vi "G#Object_GenericDefaultConstructor.vi"(0 "class path":path, 3 "control values":variant[](array[variant]), 4 "timeout in ms (-1)":i32=-1, 5 "error in (no error)":errorcluster) -> (14 "reference out":refnum<class "G#Object.lvclass">, 15 "external creator running?":bool, 19 "error out":errorcluster)   [LabVIEW 2017, in "G#Object.lvclass"]
doc: "Creates an instance of the class specified by the path by running the \"G#Object_Create.vi\" of the class. Override this construcor, else the default constructor runs. If the external create process is running, an event will be sent to let this process create and own the VI. This way LabVIEW garbage collector will not clear the object until it is destroyed or the garbage collector runs.\n\nBe careful when using this VI when building executables, since paths must be correct and make sure that all needed VIs are included in the build. Do not exclude unused dynamic dispatch VIs in the build script.\n\nNote: Will not work on RT systems."
uses:
  G#Object.lvclass
  utils/G#Object_EventType.ctl
  utils/G#Object_ObjectInfoType.ctl
  utils/G#Object_CreateMethod.ctl
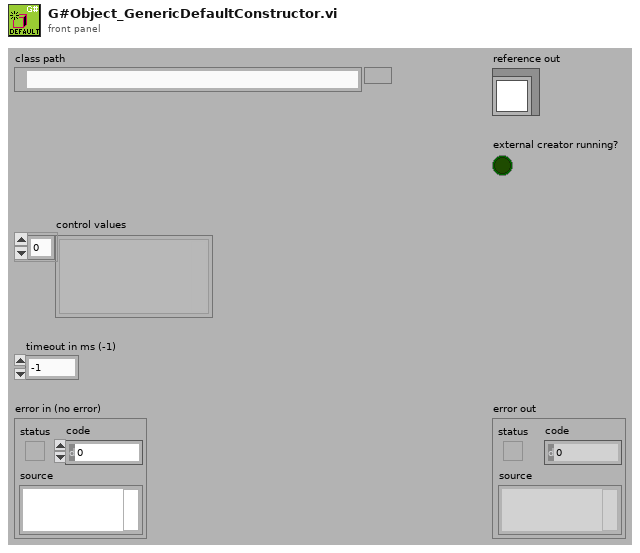
[diagram p1: front panel]
types:
  T1 = typedef "G#Object.lvclass/G#Object_ObjectInfoType.ctl" = cluster{"ObjectName":string, "ObjectID":u32, "Users":i32, "Counter":bool, "AttributeRefs":u32[], "FullClassName":string, "ClassName":string, "CreateMethod":T2, "GenericDestructorExists":bool, "Owner":string}
  T2 = typedef "G#Object.lvclass/G#Object_CreateMethod.ctl" = enum16{"Create", "Create or look up existing", "Look up existing"}
  T3 = typedef "G#Object.lvclass/G#Object_EventType.ctl" = enum16{"Created new", "Looked up existing", "Deleted", "Forced delete", "Not deleted", "Garbage collected", "Cleared", "User", "Error", "External create object", "External create class attributes", "Created class attributes", "Run constructor", "Run constructor done", "Run open method", "Run open method done"}
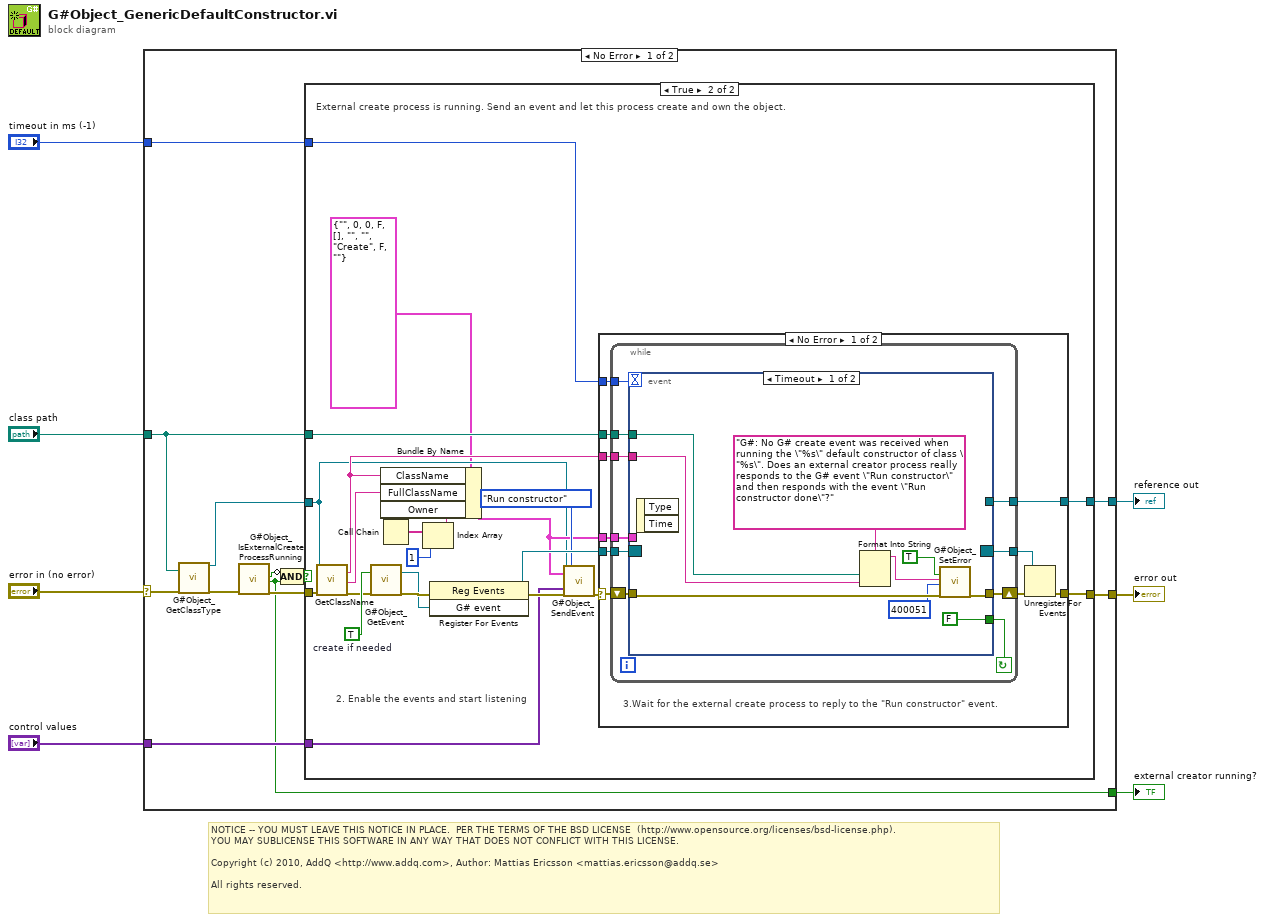
[diagram p0: block diagram]
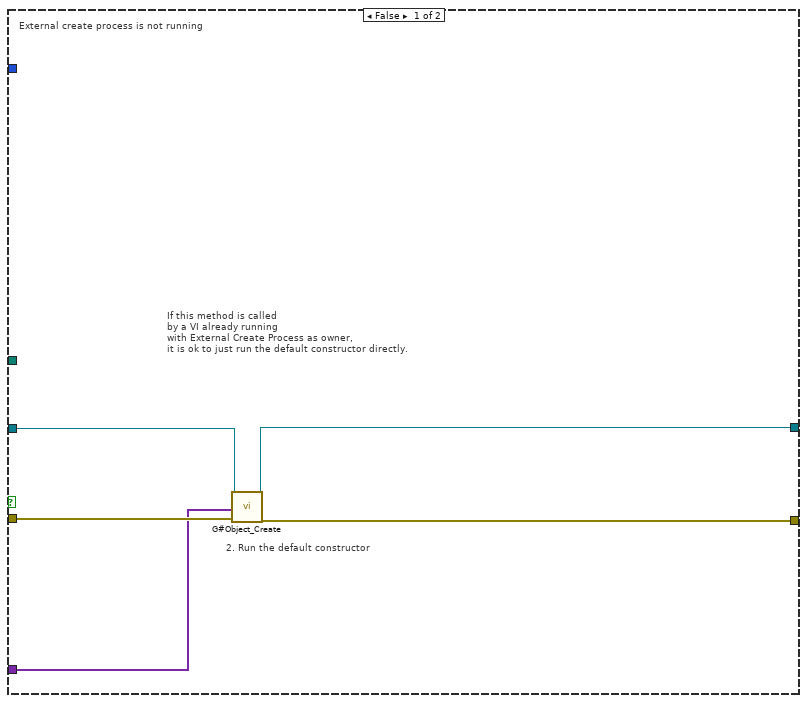
[diagram p2: hidden frame]
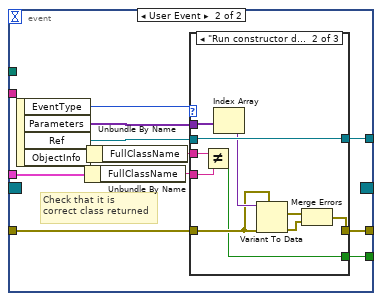
[diagram p3: hidden frame]
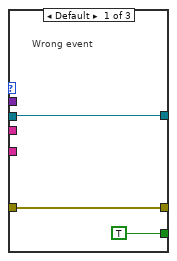
[diagram p4: hidden frame]
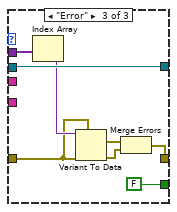
[diagram p5: hidden frame]
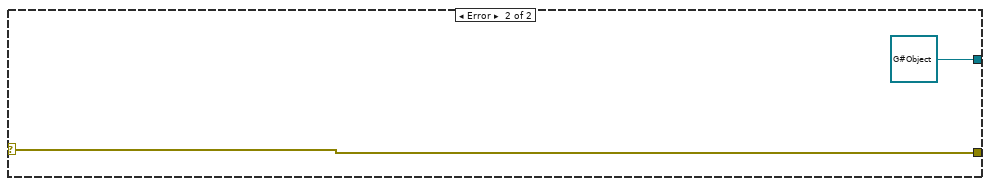
[diagram p7: hidden frame]
diagram:
  # "NOTICE -- YOU MUST LEAVE THIS NOTICE IN PLACE.  PER THE TERMS OF THE BSD LICENSE  (http://www.opensource.org/licenses/bsd-license.php).\nYOU MAY SUBLICENSE THIS SOFTWARE IN ANY WAY THAT DOES NOT CONFLICT WITH THIS LICENSE.\n\nCopyright (c) 2010, AddQ <http://www.addq.com>, Author: Mattias Ericsson <mattias.ericsson@addq.se>\n\nAll rights reserved."
  n1 = case shown="No Error" "error in (no error)" {
    selector: "error in (no error)" -> [w19 w110]
    tunnel: [w14 w110] -> w6
    tunnel: [w18 refnum<class "G#Object.lvclass"> refnum ("reference in (for type)")] -> w5
    tunnel: "control values" -> [w17 _]
    tunnel: "class path" -> [w8 _]
    tunnel: "timeout in ms (-1)" -> [w15 _]
    tunnel: [w9 _] -> w1
    frame No Error {
      n2 = call "G#Object_GetClassType.vi"("class path"=w8, "error in (no error)"=w19) -> ("reference out"=w16:refnum<class "G#Object.lvclass">, "error out"=w13:errorcluster)  [unwired: 16 in]
      n3 = call "G#Object_IsExternalCreateProcessRunning.vi"("error in (no error)"=w13) -> ("owned by external process?"=w10:bool, "external create process running?"=w9:bool, "error out"=w12:errorcluster)  [unwired: 15 in, 1 out]
      n4 = Compound Arithmetic op=AND(invert w10, w9) -> (w11:bool)
      n5 = case shown="True" w11 {
        tunnel: [w20 w44] -> w18
        tunnel: w17 -> [w21 w40]
        tunnel: w16 -> [w22 w31]
        tunnel: w15 -> [_ w37]
        tunnel: w8 -> [_ w35]
        tunnel: [w23 w29] -> w14
        tunnel: w12 -> [w24 w33]
        frame False {
          # "If this method is called\nby a VI already running\nwith External Create Process as owner,\nit is ok to just run the default constructor directly."
          # "External create process is not running"
          # "2. Run the default constructor"
          n6 = call-dynamic "G#Object_Create.vi"("reference in"=w22, "control values"=w21, "error in (no error)"=w24) -> ("reference out"=w20:refnum<class "G#Object.lvclass">, "error out"=w23:errorcluster)  [unwired: 15 in]
        }
        frame True {
          w43 = TRUE  # create if needed
          # "External create process is running. Send an event and let this process create and own the object."
          # "2. Enable the events and start listening"
          n7 = call-dynamic "GetClassName.vi"("reference in"=w31, "error in (no error)"=w33) -> ("class name"=w36:string, "full class name"=w38:string, "error out"=w34:errorcluster)  [unwired: 13 in, 2 out]
          n8 = call "G#Object_GetEvent.vi"("create if needed (T)"=w43, "error in (no error)"=w34) -> ("G# event"=w42:refnum<user-event>, "error out"=w46:errorcluster)  [unwired: 13 in, 3 out]
          n9 = Call Chain() -> (call chain=w28:string[])
          n10 = Index Array(array=w28, index=1) -> (element=w26:string)
          n11 = Bundle By Name(cluster=T1 {"ObjectName"="", "ObjectID"=0, "Users"=0, "Counter"=FALSE, "AttributeRefs"=[], "FullClassName"="", "ClassName"="", "CreateMethod"=enum."Create", "GenericDestructorExists"=FALSE, "Owner"=""} ("ObjectInfo"), "ClassName"=w36, "FullClassName"=w38, "Owner"=w26) -> (w32:T1)
          n12 = register-events(error in=w46, w42) -> (reference out=w45:refnum<event-registration>, error out=w41:errorcluster)  [unwired: 1 in]
          n13 = call "G#Object_SendEvent.vi"("reference in"=w31, "object info extended"=w32, "parameters"=w40, "error in (no error)"=w41, "G# event type"=G#Object_EventType."Run constructor") -> ("error out"=w25:errorcluster)  [unwired: 14 in]
          n14 = case shown="No Error" w25 {
            selector: w25 -> [w48 w108]
            tunnel: w45 -> [w56 _]
            tunnel: [w55 _] -> w44
            tunnel: w37 -> [w52 _]
            tunnel: w36 -> [w51 _]
            tunnel: w35 -> [w50 _]
            tunnel: w32 -> [w49 _]
            tunnel: [w47 w108] -> w29
            frame No Error {
              # "3.Wait for the external create process to reply to the \"Run constructor\" event."
              n15 = while {
                tunnel: w56 -> [w66]
                shift-right: [w64] -> w54
                shift-left: w48 -> [w65]
                tunnel: [w62] -> w55
                tunnel: [w61] -> w53
                tunnel: w52 -> [w60]
                tunnel: w51 -> [w59]
                tunnel: w50 -> [w58]
                tunnel: w49 -> [w57]
                stop <- w63 continue-if-true
                n16 = event shown="[0] Timeout" {
                  selector: w66 -> [_ _]
                  dyn-events: [_ _] -> w61
                  timeout: w60 -> [_ _]
                  tunnel: w65 -> [w73 w85]
                  tunnel: [w74 w82] -> w64
                  tunnel: [FALSE w81] -> w63
                  tunnel: [_ w80] -> w62
                  tunnel: w59 -> [w68 _]
                  tunnel: w58 -> [w69 _]
                  tunnel: w57 -> [_ w77]
                  event Timeout {
                    n17 = event-data() -> ()  [unwired: 1 in, 2 out]
                    n18 = Format Into String(format string="G#: No G# create event was received when running the \"%s\" default constructor of class \"%s\". Does an external creator process really responds to the G# event \"Run constructor\" and then responds with the event \"Run constructor done\"?" ("source"), w69, w68) -> (resulting string=w70:string)  [unwired: 2 in, 1 out]
                    n19 = call "G#Object_SetError.vi"("error (F)"=TRUE ("error"), "source"=w70, "code"=400051, "error in (no error)"=w73) -> ("error out"=w74:errorcluster)  [unwired: 15 in]
                  }
                  event User Event {
                    # "Check that it is\ncorrect class returned"
                    n20 = event-data() -> ("EventType"=w86:T3, "Parameters"=w84:variant[], "Ref"=w83:refnum<class "G#Object.lvclass">, "ObjectInfo"=w79:T1)  [unwired: 1 in]
                    n21 = Unbundle By Name(w77) -> ("FullClassName"=w76:string)
                    n22 = Unbundle By Name(w79) -> ("FullClassName"=w78:string)
                    n23 = case shown="\"Run constructor done\"" w86 {
                      tunnel: w85 -> [w88 w96 w104]
                      tunnel: w84 -> [_ w98 w106]
                      tunnel: w83 -> [w89 w99 w107]
                      tunnel: [w88 w92 w102] -> w82
                      tunnel: [TRUE w94 FALSE] -> w81
                      tunnel: [w89 w99 w107] -> w80
                      tunnel: w78 -> [_ w95 _]
                      tunnel: w76 -> [_ w90 _]
                      frame Default {
                        # "Wrong event"
                      }
                      frame "Run constructor done" {
                        n24 = Not Equal?(x=w95, y=w90) -> (x != y?=w94:bool)
                        n25 = Index Array(array=w98) -> (element=w97:variant)  [unwired: 1 in]
                        n26 = Variant To Data(error in=w96, type=w96, Variant=w97) -> (data=w91:errorcluster, error out=w93:errorcluster)
                        n27 = Merge Errors(w91, w93) -> (w92:errorcluster)
                      }
                      frame "Error" {
                        n28 = Index Array(array=w106) -> (element=w105:variant)  [unwired: 1 in]
                        n29 = Variant To Data(error in=w104, type=w104, Variant=w105) -> (data=w101:errorcluster, error out=w103:errorcluster)
                        n30 = Merge Errors(w101, w103) -> (w102:errorcluster)
                      }
                    }
                  }
                }
              }
              n31 = Unregister For Events(event registration refnum=w53, error in=w54) -> (error out=w47:errorcluster)
            }
            frame Error {
            }
          }
        }
      }
    }
    frame Error {
    }
  }
  "error out" <- w6
  "reference out" <- w5
  "external creator running?" <- w1
